vi "Initialize.vi"(8 "error in (no error)":errorcluster, 11 "SubPanel Actor in":refnum<class "SubPanel Actor.lvclass">) -> (0 "error out":errorcluster, 3 "SubPanel Actor out":refnum<class "SubPanel Actor.lvclass">)   [LabVIEW 2020, in "SubPanel Actor.lvlib" / "SubPanel Actor.lvclass"]
uses:
  SubPanel Actor.lvclass
  SubPanel Actor.lvclass/SubPanel Actor.ctl
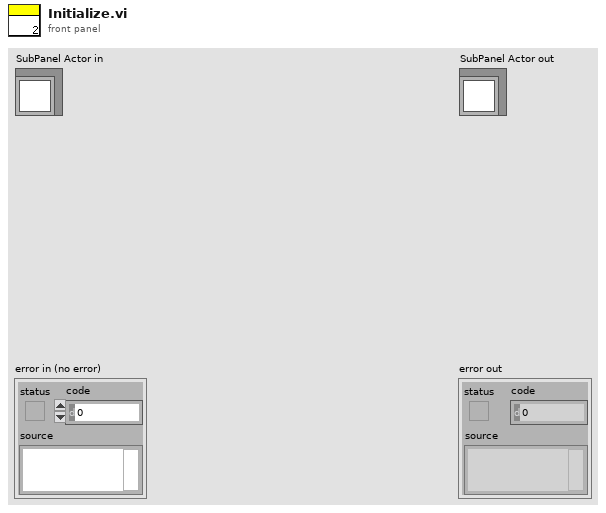
[diagram p1: front panel]
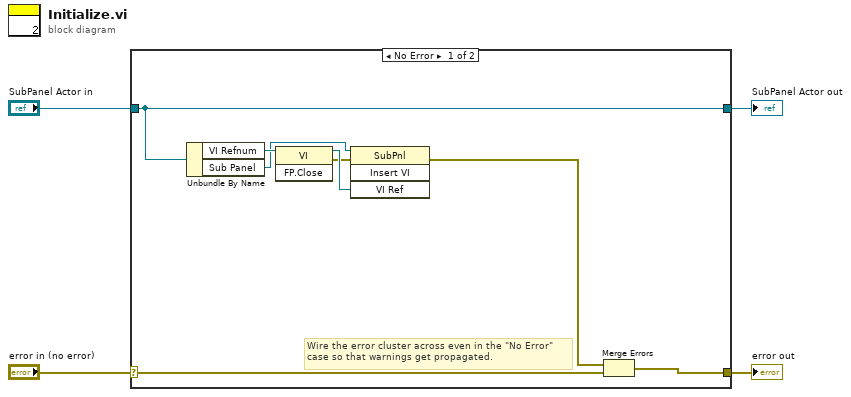
[diagram p0: block diagram]
diagram:
  n1 = case shown="No Error" "error in (no error)" {
    selector: "error in (no error)" -> [w12 w14]
    tunnel: [w7 w14] -> w3
    tunnel: [w11 w13] -> w1
    tunnel: "SubPanel Actor in" -> [w11 w13]
    frame No Error {
      # "Wire the error cluster across even in the \"No Error\"\ncase so that warnings get propagated."
      n2 = Unbundle By Name(w11) -> ("VI Refnum"=w10:refnum<vi>, "Sub Panel"=w9:refnum<vi>)
      n3 = invoke class="VI" method="FP.Close"(reference=w10) -> (reference out=w8:refnum<vi>, error out=w5:errorcluster)  [unwired: 2 in, 1 out]
      n4 = invoke class="SubPnl" method="Insert VI"(reference=w9, error in=w5, "VI Ref"=w8) -> (error out=w6:errorcluster)  [unwired: 1 in, 3 out]
      n5 = Merge Errors(w6, w12) -> (w7:errorcluster)
    }
    frame Error {
    }
  }
  "error out" <- w3
  "SubPanel Actor out" <- w1
